vi "Untitled 3.vi"() -> ()   [LabVIEW 2022 SP3]
panel:
  out "standard output":string
  in  "command line":string
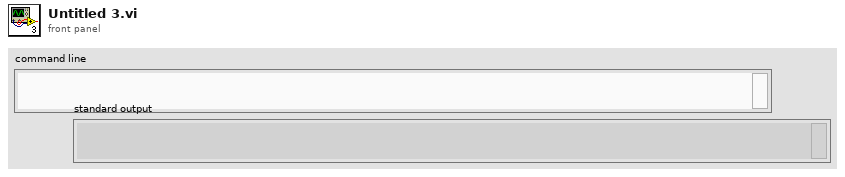
[diagram p1: front panel]
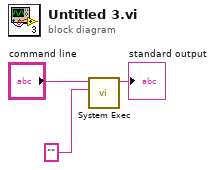
[diagram p0: block diagram]
diagram:
  n1 = call <vilib>:"System Exec.vi"("standard input"="", "command line"="command line") -> ("standard output"=→"standard output":string)  [unwired: 6 in, 3 out]
